vi "enqueue_message.vi"(6 "Priority Message? (F)":bool caption="优先消息？(F)", 8 "error in (no error)":errorcluster caption="错误输入（无错误）", 9 "Message Data":variant caption="消息数据", 10 "Message":string caption="消息", 11 "Message Queue":refnum<queue> caption="消息队列") -> (0 "error out":errorcluster caption="错误输出", 3 "dup Message Queue":refnum<queue> caption="消息队列副本")   [LabVIEW 2015, in "message_queue.lvlib"]
doc: "对于标准消息，将消息加入队列。对于优先消息，将消息加入队列的头部。"
uses:
  message_queue.lvlib
  message_cluster.ctl
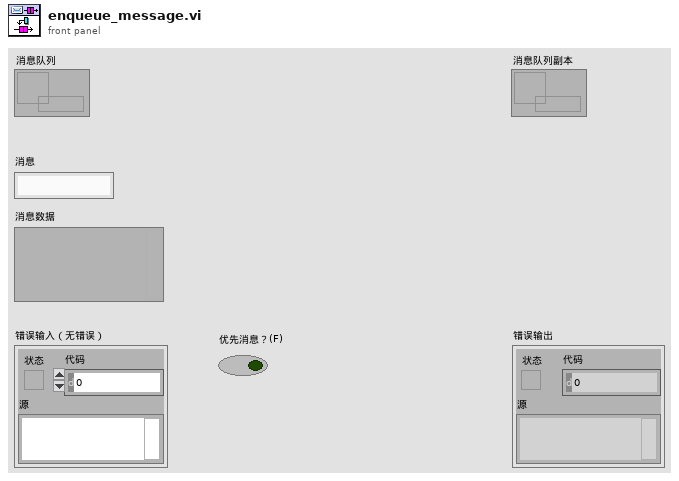
[diagram p1: front panel]
types:
  T1 = typedef "message_queue.lvlib/message_cluster.ctl" = cluster{"Message":string, "Message Data":variant}
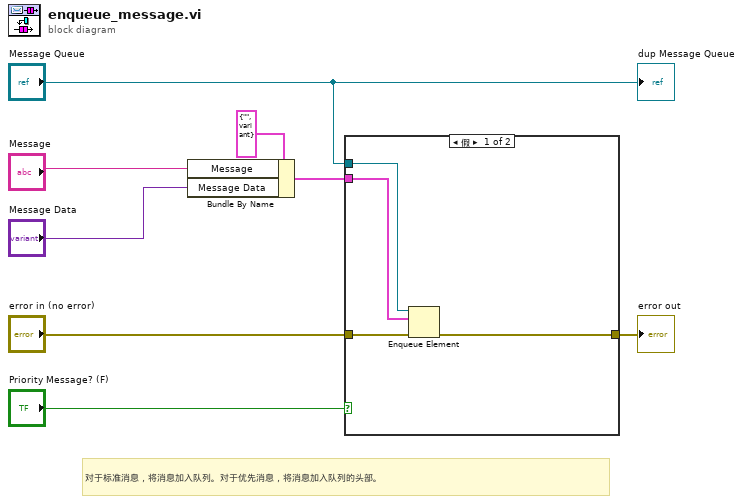
[diagram p0: block diagram]
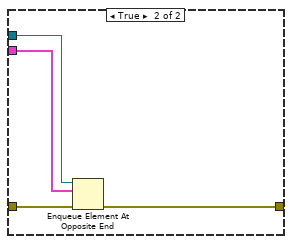
[diagram p2: hidden frame]
diagram:
  # "对于标准消息，将消息加入队列。对于优先消息，将消息加入队列的头部。"
  n1 = Bundle By Name(cluster=T1 {"Message"="", "Message Data"=variant} ("Message Cluster"), "Message"="Message", "Message Data"="Message Data") -> (w1:T1)
  n2 = case shown="假" "Priority Message? (F)" {
    tunnel: "error in (no error)" -> [w12 w16]
    tunnel: [w11 w15] -> w3
    tunnel: "Message Queue" -> [w10 w14]
    tunnel: w1 -> [w9 w13]
    frame False {
      n3 = Enqueue Element(queue=w10, element=w9, error in (no error)=w12) -> (error out=w11:errorcluster)  [unwired: 1 in, 2 out]
    }
    frame True {
      n4 = Enqueue Element At Opposite End(queue=w14, element=w13, error in (no error)=w16) -> (error out=w15:errorcluster)  [unwired: 1 in, 2 out]
    }
  }
  "error out" <- w3
  "dup Message Queue" <- "Message Queue"
